vi "Inverse_Kinematics.vi"(9 "Numeric in":dbl, 10 "Numeric 3":dbl, 11 "Colors in":T1={"Base"=16750848, "Link 1"=16764006, "Joint 2"=26316, "Link 2"=6723993, "EOF"=16724787}) -> (1 "Picture Out":picture, 2 "Angle 3":dbl, 3 "Angle 4":dbl, 4 "angle2":dbl, 5 "Numeric out":dbl)   [LabVIEW 2024]
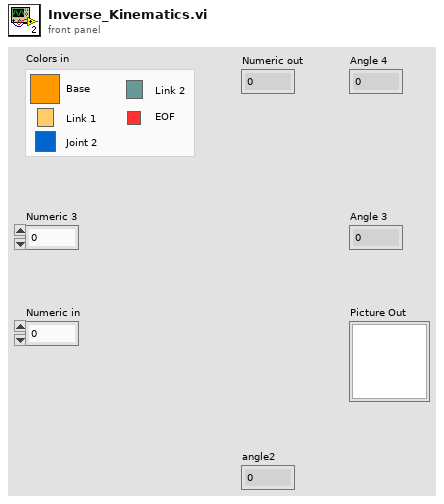
[diagram p1: front panel]
types:
  T1 = cluster{"Base":u32, "Link 1":u32, "Joint 2":u32, "Link 2":u32, "EOF":u32}
  T2 = cluster{"top":dbl, "left":dbl, "height":dbl, "width":dbl}
  T3 = cluster{"left":dbl, "top":dbl, "right":dbl, "bottom":dbl}
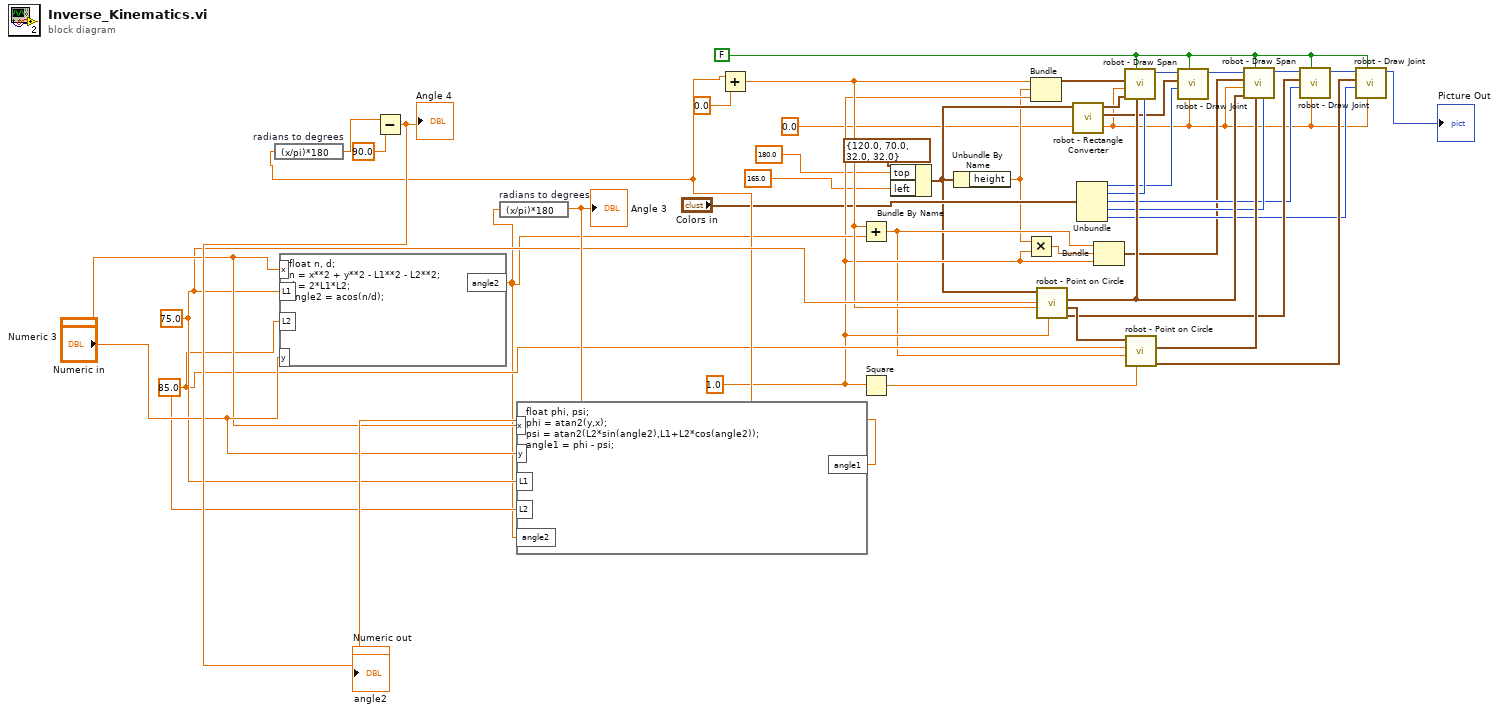
[diagram p0: block diagram]
diagram:
  w39 = 75.0 ("Length 7")
  w33 = 85.0 ("Length 8")
  w30 = 1.0 ("Scale Factor")
  w28 = FALSE ("Add details")
  w1 = 0.0 ("Light Direction")
  n1 = formula code="float n, d;\nn = x**2 + y**2 - L1**2 - L2**2;\nd = 2*L1*L2;\nangle2 = acos(n/d);"("x"="Numeric 3", "y"="Numeric in", "L1"=w39, "L2"=w33) -> ("angle2"=w32:dbl)
  n2 = expression code="(x/pi)*180" "radians to degrees"(w32) -> (→"Angle 3" →"angle2":dbl)
  n3 = formula code="float phi, psi;\nphi = atan2(y,x);\npsi = atan2(L2*sin(angle2),L1+L2*cos(angle2));\nangle1 = phi - psi;"("x"="Numeric 3", "y"="Numeric in", "L1"=w39, "L2"=w33, "angle2"=w32) -> ("angle1"=w34:dbl)
  n4 = expression code="(x/pi)*180" "radians to degrees"(w34) -> (w36:dbl)
  n5 = Subtract(x=w36, y=90.0) -> (x-y=→"Angle 4" →"Numeric out":dbl)
  n6 = Add(x=w34, y=0.0) -> (x+y=w35:dbl)
  n7 = Add(x=w35, y=w32) -> (x+y=w29:dbl)
  n8 = Square(x=w30) -> (x^2=w19:dbl)
  n9 = Bundle By Name(cluster=T2 {"top"=120.0, "left"=70.0, "height"=32.0, "width"=32.0} ("Circle"), "top"=180.0 ("Base position Y"), "left"=165.0 ("Base position X")) -> (w17:T2)
  n10 = Unbundle By Name(w17) -> ("height"=w5:dbl)
  n11 = Multiply(x=w5, y=w30) -> (x*y=w2:dbl)
  n12 = Bundle(w35, "height"=w5, "Scale Factor"=w30) -> (w4:cluster{dbl, "height":dbl, "Scale Factor":dbl})  [unwired: 1 in]
  n13 = call "robot - Point on Circle.vi"("Scale Factor"=w30, "Angle"=w35, "Radius"=w39, "Rect In"=w17) -> ("Scaled Rect Out"=w22:T3, "Rect Out"=w23:T3, "scaled point"=w21:cluster{"x":dbl, "y":dbl})  [unwired: 4 in, 1 out]
  n14 = call "robot - Rectangle Converter.vi"("Rect"=w17) -> ("Rect Out"=w11:T3, "Center"=w18:cluster{"x":dbl, "y":dbl})  [unwired: 9 in]
  n15 = Unbundle("Colors in") -> ("Base"=w10:u32, "Link 1"=w12:u32, "Joint 2"=w9:u32, "Link 2"=w13:u32, "EOF"=w8:u32)
  n16 = Bundle(w29, w2, "Scale Factor"=w30) -> (w3:cluster{dbl, dbl, "Scale Factor":dbl})  [unwired: 1 in]
  n17 = call "robot - Draw Span.vi"("Color"=w12, "Center 2"=w21, "Enhance Style"=w28, "Center 1"=w18, "Light Direction"=w1, "Circle Spec"=w4) -> ("Picture Out"=w7:picture)  [unwired: 5 in]
  n18 = call "robot - Point on Circle.vi"("Scale Factor"=w19, "Angle"=w29, "Radius"=w33, "Rect In"=w23) -> ("Scaled Rect Out"=w20:T3, "scaled point"=w24:cluster{"x":dbl, "y":dbl})  [unwired: 4 in, 2 out]
  n19 = call "robot - Draw Joint.vi"("Light Direction"=w1, "Enhance Style"=w28, "Color"=w10, "Rectangle"=w11, "Picture In"=w7) -> ("Picture Out"=w25:picture)  [unwired: 6 in]
  n20 = call "robot - Draw Span.vi"("Color"=w13, "Center 2"=w24, "Enhance Style"=w28, "Center 1"=w21, "Light Direction"=w1, "Circle Spec"=w3, "Picture In"=w25) -> ("Picture Out"=w6:picture)  [unwired: 4 in]
  n21 = call "robot - Draw Joint.vi"("Light Direction"=w1, "Enhance Style"=w28, "Color"=w9, "Rectangle"=w22, "Picture In"=w6) -> ("Picture Out"=w26:picture)  [unwired: 6 in]
  n22 = call "robot - Draw Joint.vi"("Light Direction"=w1, "Enhance Style"=w28, "Color"=w8, "Rectangle"=w20, "Picture In"=w26) -> ("Picture Out"=→"Picture Out":picture)  [unwired: 6 in]
